vi "Interactive Update System Log.vi"(0 "Previous Step":i32[](array[numeric]), 1 "Current Step in":i32, 2 "Name for Value":string, 3 "Test Value":dbl, 5 "Next Step":i32[](array[numeric]), 9 "Button Press":i32, 11 "error in (no error)":errorcluster, 12 "Report Info":T1[](array[typedef]), 13 "Log Value":dbl[](array[numeric])) -> (4 "End of SubTest?":bool, 6 "Current Step out":i32, 10 "Update Log/Config Ctrls?":bool, 15 "error out":errorcluster)   [LabVIEW 2018, in "Controller (Host).lvlib"]
uses:
  Controller (Host).lvlib
  File IO/File IO.lvlib
  Testing UI 1/Testing UI 1.lvlib
  File IO/Public Controls/Report Sheet Names.ctl
  File IO/Public Controls/Write to Report.ctl
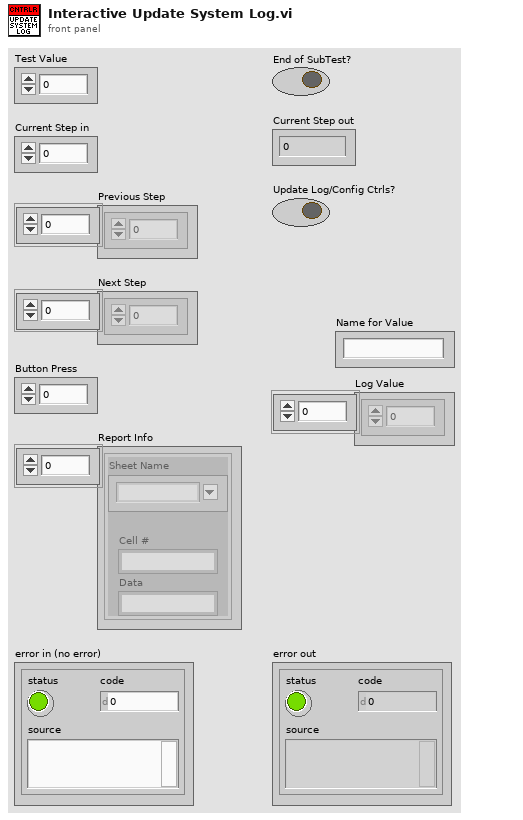
[diagram p1: front panel]
types:
  T1 = typedef "File IO.lvlib/Write to Report.ctl" = cluster{"Sheet Name":T2, "Cell #":string, "Data":string}
  T2 = typedef "File IO.lvlib/Report Sheet Names.ctl" = string
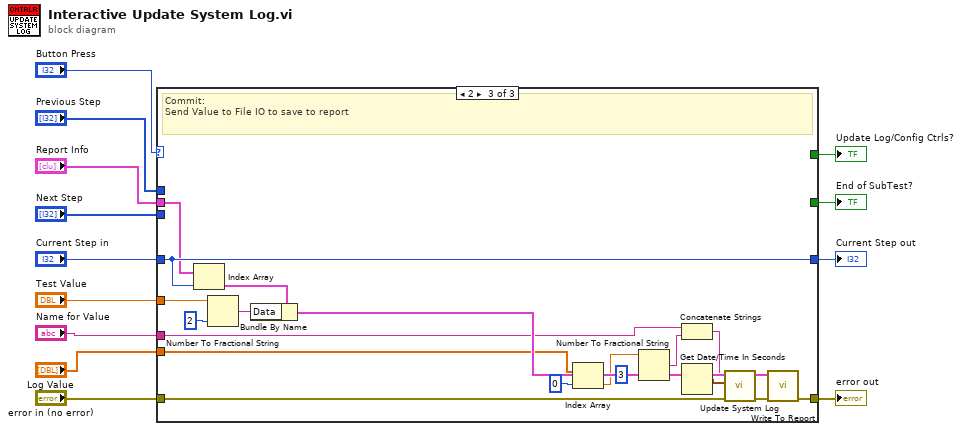
[diagram p0: block diagram]
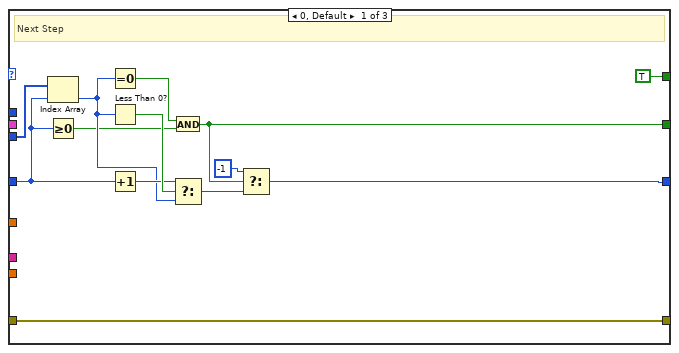
[diagram p2: hidden frame]
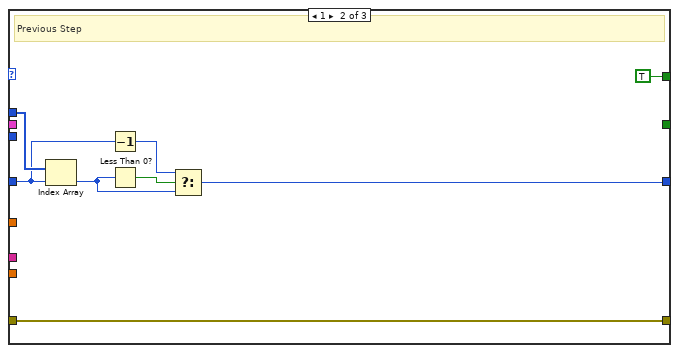
[diagram p3: hidden frame]
diagram:
  n1 = case shown="2" "Button Press" {
    tunnel: "Current Step in" -> [w15 w27 w51]
    tunnel: [w17 w29 w51] -> w10
    tunnel: "Next Step" -> [w25 _ _]
    tunnel: [TRUE TRUE _] -> w11
    tunnel: "Previous Step" -> [_ w34 _]
    tunnel: "Test Value" -> [_ _ w49]
    tunnel: "error in (no error)" -> [w22 w28 w43]
    tunnel: [w22 w28 w52] -> w9
    tunnel: [w16 _ _] -> w12
    tunnel: "Report Info" -> [_ _ w45]
    tunnel: "Log Value" -> [_ _ w36]
    tunnel: "Name for Value" -> [_ _ w35]
    frame 0, Default {
      # "Next Step"
      n2 = Index Array(array=w25, index=w15) -> (element=w21:i32)
      n3 = Greater Or Equal To 0?(x=w15) -> (x >= 0?=w14:bool)
      n4 = Equal To 0?(x=w21) -> (x = 0?=w19:bool)
      n5 = Less Than 0?(x=w21) -> (x < 0?=w24:bool)
      n6 = Increment(x=w15) -> (x+1=w23:i32)
      n7 = And(x=w19, y=w14) -> (x .and. y?=w16:bool)
      n8 = Select(t=w23, s=w24, f=w21) -> (s? t:f=w20:i32)
      n9 = Select(t=-1, s=w16, f=w20) -> (s? t:f=w17:i32)
    }
    frame 1 {
      # "Previous Step"
      n10 = Index Array(array=w34, index=w27) -> (element=w31:i32)
      n11 = Decrement(x=w27) -> (x-1=w30:i32)
      n12 = Less Than 0?(x=w31) -> (x < 0?=w32:bool)
      n13 = Select(t=w30, s=w32, f=w31) -> (s? t:f=w29:i32)
    }
    frame 2 {
      # "Commit:\nSend Value to File IO to save to report"
      n14 = Index Array(array=w45, index=w51) -> (element=w50:T1)
      n15 = Number To Fractional String(number=w49, precision (6)=i16 2) -> (F-format string=w48:string)  [unwired: 2 in]
      n16 = Bundle By Name(cluster=w50, "Data"=w48) -> (w47:T1)
      n17 = Index Array(array=w36, index=0) -> (element=w39:dbl)
      n18 = Number To Fractional String(number=w39, precision (6)=i16 3) -> (F-format string=w38:string)  [unwired: 2 in]
      n19 = Concatenate Strings(w35, w38) -> (w41:string)
      n20 = Get Date/Time In Seconds() -> (seconds since 1Jan1904=w40:timestamp)
      n21 = call "Update System Log.vi"("error in (no error)"=w43, 10:w40, "Message"=w41) -> ("error out"=w42:errorcluster)  [unwired: 8 in]
      n22 = call "Write To Report.vi"("error in (no error)"=w42, "Report Info"=w47) -> ("error out"=w52:errorcluster)  [unwired: 9 in]
    }
  }
  "End of SubTest?" <- w12
  "Update Log/Config Ctrls?" <- w11
  "Current Step out" <- w10
  "error out" <- w9
